vi "Update Last Comm Time.vi"(8 "error in (no error)":errorcluster, 11 "Network Info in":T1 {"Last Comm Time" format="%<%H:%M:%S%3u\n%Y/%m/%d>T"; "Remote Port" format="%.0x"}) -> (0 "error out":errorcluster, 3 "Network Info out":T1 {"Last Comm Time" format="%<%H:%M:%S%3u\n%Y/%m/%d>T"; "Remote Port" format="%.0x"})   [LabVIEW 2022 SP3]
doc: "Author: Scott Hannahs <sth@magnet.fsu.edu>\nCopyright 2018 Florida State University, All rights reserved."
uses:
  RT Controls/Network Info.ctl
  RT Controls/RT System Auth Level.ctl
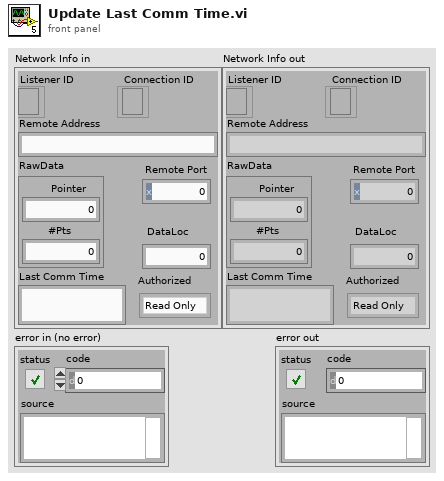
[diagram p1: front panel]
types:
  T1 = typedef "Network Info.ctl" = cluster{"Listener ID":refnum<k5>, "Connection ID":refnum<k5>, "Remote Address":string, "Remote Port":u16, "DataLoc":u32, "RawData":cluster{"#Pts":u32, "Pointer":u32}, "Last Comm Time":timestamp, "Authorized":T2}
  T2 = typedef "RT System Auth Level.ctl" = enum16{"Read Only", "Operator", "Admin"}
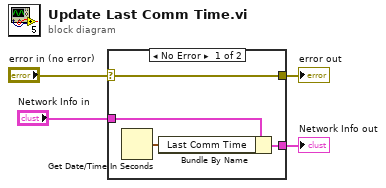
[diagram p0: block diagram]
diagram:
  n1 = case shown="No Error" "error in (no error)" {
    selector: "error in (no error)" -> [w7 w10]
    tunnel: [w7 w10] -> w4
    tunnel: [w6 w9] -> w2
    tunnel: "Network Info in" -> [w5 w9]
    frame No Error {
      n2 = Get Date/Time In Seconds() -> (seconds since 1Jan1904=w8:timestamp)
      n3 = Bundle By Name(cluster=w5, "Last Comm Time"=w8) -> (w6:T1)
    }
    frame Error {
    }
  }
  "error out" <- w4
  "Network Info out" <- w2
